vi "Update Interface.vi"(8 "error in (no error)":errorcluster, 9 "Payload (Optional)":variant, 10 "UI update option":T1(ring)) -> (0 "error out":errorcluster)   [LabVIEW 2018, in "Tracker Main.lvlib"]
doc: "Updates interface according to the latest updates in the setting file.\n_____\nCreated using Delacor QMH Event Scripter 4.2.1.88."
uses:
  Tracker Main.lvlib
  Update Interface Argument--cluster.ctl
  Private API/Typedefs/CTL_UI_Update_Option.ctl
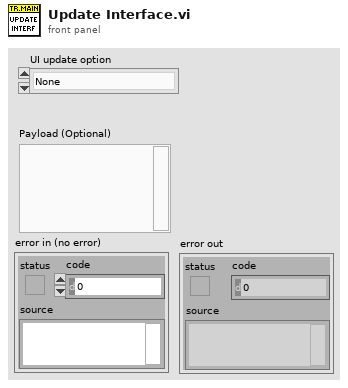
[diagram p1: front panel]
types:
  T1 = enum16{"None", "Set state 01 (SW Init)", "Update IO indicator", "Update Conditions indicator", "Set state 02 (Unlock UI)"}
  T2 = typedef "Tracker Main.lvlib/Update Interface Argument--cluster.ctl" = cluster{"UI update option":T3}
  T3 = typedef "Tracker Main.lvlib/CTL_UI_Update_Option.ctl" = cluster{"UI update option":enum16{"None", "Set state 01 (SW Init)", "Update IO indicator", "Update Conditions indicator", "Set state 02 (Unlock UI)"}, "Payload (Optional)":variant}
  T4 = typedef "Tracker Main.lvlib/Request Events--cluster.ctl" = cluster{"Stop Module":refnum<user-event>, "Show Panel":refnum<user-event>, "Hide Panel":refnum<user-event>, "Get Module Execution Status":refnum<user-event>, "Show Diagram":refnum<user-event>, "SW Init":refnum<user-event>, "Prepare to Exit":refnum<user-event>, "Update Status and History":refnum<user-event>, "Update Interface":refnum<user-event>, "HW Init":refnum<user-event>, "Load Minimal Set of Modules":refnum<user-event>, "Update Cage Layout":refnum<user-event>, "HW Init Outcome check":refnum<user-event>, "Switch Offline":refnum<user-event>}
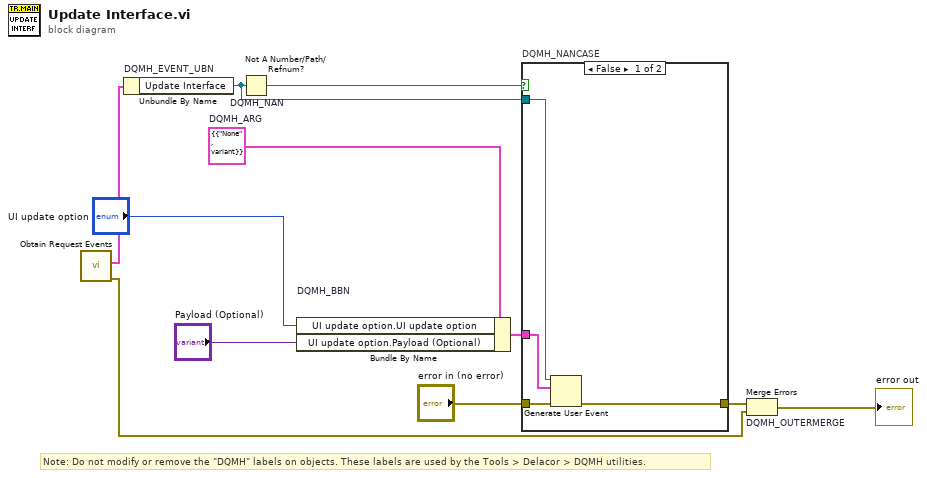
[diagram p0: block diagram]
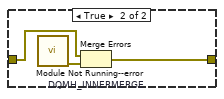
[diagram p2: hidden frame]
diagram:
  w5 = T2 {"UI update option"={"UI update option"=enum."None", "Payload (Optional)"=variant}}  # DQMH_ARG
  # "Note: Do not modify or remove the \"DQMH\" labels on objects. These labels are used by the Tools > Delacor > DQMH utilities."
  n1 = call "Obtain Request Events.vi"() -> ("error out"=w4:errorcluster, "Tracker Main Request Events"=w3:T4)  [unwired: 10 in]
  n2 = Unbundle By Name "DQMH_EVENT_UBN"(w3) -> ("Update Interface"=w7:refnum<user-event>)
  n3 = Not A Number/Path/Refnum? "DQMH_NAN"(number/path/refnum=w7) -> (NaN/Path/Refnum?=w8:bool)
  n4 = Bundle By Name "DQMH_BBN"(cluster=w5, "UI update option.UI update option"="UI update option", "UI update option.Payload (Optional)"="Payload (Optional)") -> (w9:T2)
  n5 = case "DQMH_NANCASE" shown="False" w8 {
    tunnel: "error in (no error)" -> [w15 w18]
    tunnel: [w14 w17] -> w6
    tunnel: w7 -> [w13 _]
    tunnel: w9 -> [w12 _]
    frame False {
      n6 = Generate User Event(user event=w13, event data cluster=w12, error in=w15) -> (error out=w14:errorcluster)  [unwired: 1 in, 1 out]
    }
    frame True {
      n7 = call "Module Not Running--error.vi"() -> ("error out"=w16:errorcluster)  [unwired: 11 in]
      n8 = Merge Errors "DQMH_INNERMERGE"(w18, w16) -> (w17:errorcluster)
    }
  }
  n9 = Merge Errors "DQMH_OUTERMERGE"(w6, w4) -> (→"error out":errorcluster)
